vi "Tell Child.vi"(4 "Priority":bool, 6 "rUID":string, 7 "Actor in":refnum<class "Actor.lvclass">, 8 "Error in":errorcluster) -> (0 "Error out":errorcluster, 5 "Actor out":refnum<class "Actor.lvclass">)   [LabVIEW 2020, in "jettl.lvlib" / "Start jettl Msg.lvlib" / "Start.lvlib"]
doc: "jettl 6.14.1.98\nNathan Davis - Nathan Davis\nCopyright (c) 2026, Nathan Davis\nMIT"
uses:
  Start.lvlib
  Actor/Actor.lvclass
  jettl.lvlib
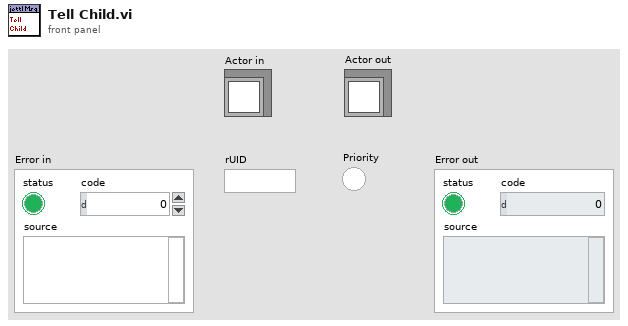
[diagram p1: front panel]
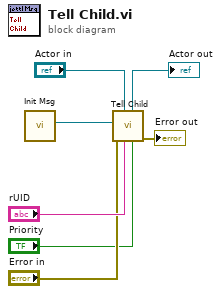
[diagram p0: block diagram]
diagram:
  n1 = call "Init Msg.vi"() -> ("Msg"=w2:refnum<class "Msg.lvclass">)  [unwired: 11 in]
  n2 = call "Tell Child.vi"("Priority"="Priority", "UID"="rUID", "Actor in"="Actor in", "Error in"="Error in", "Msg"=w2) -> ("Error out"=→"Error out":errorcluster, "Actor out"=→"Actor out":refnum<class "Actor.lvclass">)  [unwired: 5 in]
